vi "Serial Test.vi"() -> ()   [LabVIEW 2013]
uses:
  Program Files (x86)/National Instruments/LabVIEW 2013/examples/Instrument IO/Serial/support/Serial - Settings.ctl
  <vilib>/Instr/_visa.llb/VISA Configure Serial Port (Instr).vi
panel:
  in  "불리언":bool
  out "숫자형":i32=1422
  in  "버퍼 쓰기":string="L100nM100nR100nn"
  in  "정지":bool
  in  "Serial Settings":T1={"baud rate"=2400, "data bits"=8, "parity"=enum."None", "stop bits"=10, "flow control"=0} {"flow control" items=["None"=0, "XON/XOFF"=1, "RTS/CTS"=2, "DTR/DSR"=4]; "stop bits" items=["1.0"=10, "1.5"=15, "2.0"=20]; "data bits" min=5 max=8 step=1; "baud rate" items=["75"=75, "110"=110, "134"=134, "150"=150, "300"=300, "600"=600, "1200"=1200, "1800"=1800, "2400"=2400, "4800"=4800, "7200"=7200, "9600"=9600, "14400"=14400, "19200"=19200, "28800"=28800, "38400"=38400, "56000"=56000, "57600"=57600, "115200"=115200, "128000"=128000, "230400"=230400]}
  out "bytes read":u32=37
  out "Response":string
  in  "delay before read (ms)":u32=80
  in  "VISA resource name":refnum<visa-resource-name>="COM3"
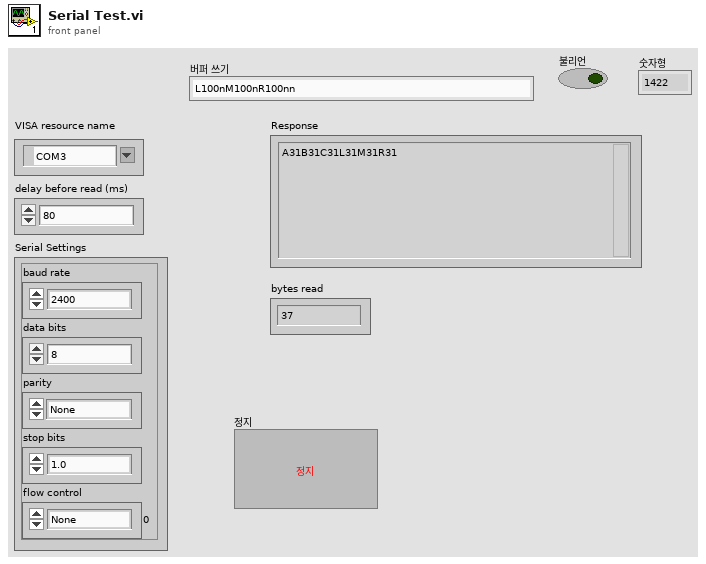
[diagram p1: front panel]
types:
  T1 = typedef "Serial - Settings.ctl" = cluster{"baud rate":u32, "data bits":u16, "parity":enum16{"None", "Odd", "Even", "Mark", "Space"}, "stop bits":u16, "flow control":u16}
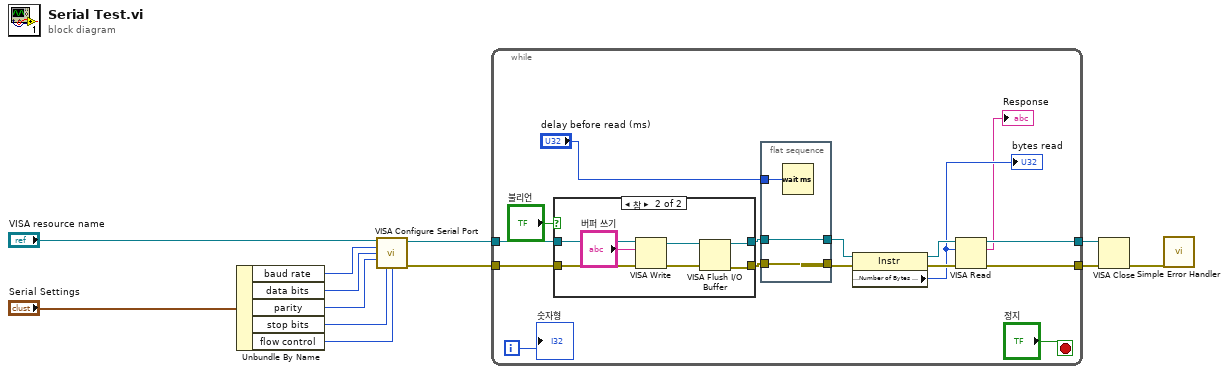
[diagram p0: block diagram]
diagram:
  n1 = Unbundle By Name("Serial Settings") -> ("baud rate"=w5:u32, "data bits"=w4:u16, "parity"=w3:enum16{"None", "Odd", "Even", "Mark", "Space"}, "stop bits"=w2:u16, "flow control"=w1:u16)
  n2 = call-poly "VISA Configure Serial Port"("VISA resource name"="VISA resource name", "baud rate (9600)"=w5, "data bits (8)"=w4, "parity (0:none)"=w3, "stop bits (10: 1 bit)"=w2, "flow control (0:none)"=w1) -> ("VISA resource name out"=w10:refnum<visa-resource-name>, "error out"=w11:errorcluster)  [unwired: 3 in, 5 out]
  n3 = while {
    tunnel: w11 -> [w28]
    tunnel: w10 -> [w27]
    tunnel: [w26] -> w9
    tunnel: [w25] -> w8
    i -> [w16]
    stop <- "정지" stop-if-true
    n4 = case shown="참" "불리언" {
      tunnel: w28 -> [w29 w37]
      tunnel: w27 -> [w30 w36]
      tunnel: [w29 w34] -> w24
      tunnel: [w30 w31] -> w22
      frame False {
      }
      frame True {
        n5 = VISA Write(VISA resource name=w36, write buffer="버퍼 쓰기", error in (no error)=w37) -> (VISA resource name out=w33:refnum<visa-resource-name>, error out=w32:errorcluster)  [unwired: 1 out]
        n6 = VISA Flush I/O Buffer(VISA resource name=w33, error in (no error)=w32) -> (VISA resource name out=w31:refnum<visa-resource-name>, error out=w34:errorcluster)  [unwired: 1 in]
      }
    }
    n7 = flat-sequence {
      tunnel: w24 -> [w39]
      tunnel: [w39] -> w23
      tunnel: w22 -> [w38]
      tunnel: [w38] -> w21
      tunnel: "delay before read (ms)" -> [w40]
      frame #0 {
        n8 = Wait (ms)(milliseconds to wait=w40) -> ()  [unwired: 1 out]
      }
    }
    n9 = property class="Instr"(reference=w21, error in=w23) -> (reference out=w20:refnum<visa-resource-name>, error out=w19:errorcluster, "Serial Settings:Number of Bytes at Serial Port"=w18:u32)
    "bytes read" <- w18
    n10 = VISA Read(VISA resource name=w20, byte count=w18, error in (no error)=w19) -> (VISA resource name out=w25:refnum<visa-resource-name>, read buffer=→"Response":string, error out=w26:errorcluster)  [unwired: 1 out]
    "숫자형" <- w16
  }
  n11 = VISA Close(VISA resource name=w8, error in (no error)=w9) -> (error out=w7:errorcluster)
  n12 = call <vilib>:"Simple Error Handler.vi"("error in (no error)"=w7) -> ()  [unwired: 1 in, 8 out]
